vi "GetFilePathAndDate.vi"(8 "error in (no error)":errorcluster, 9 "String":string, 10 "Index":i32, 11 "Path":path) -> (0 "error out":errorcluster, 2 "creation date":u32, 3 "file out":path)   [LabVIEW 2015]
uses:
  <userlib>/_OpenG.lib/file/file.llb/File Info Record__ogtk.ctl
panel:
  out "file info":T1={"type"="????", "creator"="????", "permissions"=438, "data size"=5687, "res size"=0, "creation date"=3188231670, "modification date"=3188232972, "bFolder"=FALSE, "bInvisible"=FALSE, "location"={"vertical"=0, "horizontal"=0}, "owner"="", "group"=""} {"modification date" format="%<%H:%M:%S\n%m/%d/%Y>T"; "creation date" format="%<%H:%M:%S\n%m/%d/%Y>T"; "permissions" format="%.0x"}
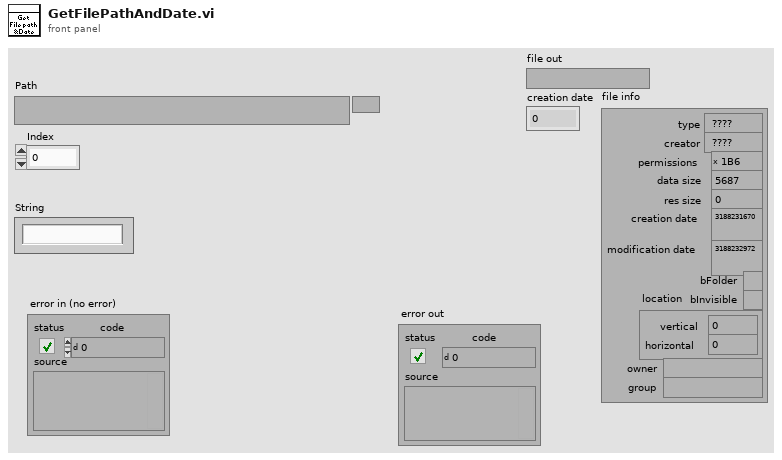
[diagram p1: front panel]
types:
  T1 = typedef "File Info Record__ogtk.ctl" = cluster{"type":string, "creator":string, "permissions":i32, "data size":i32, "res size":i32, "creation date":u32, "modification date":u32, "bFolder":bool, "bInvisible":bool, "location":cluster{"vertical":i16, "horizontal":i16}, "owner":string, "group":string}
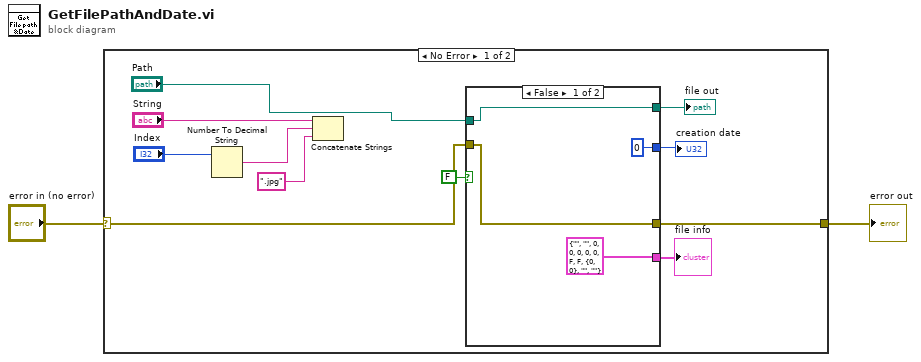
[diagram p0: block diagram]
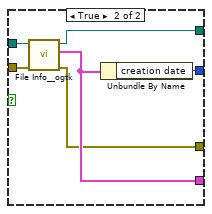
[diagram p2: hidden frame]
diagram:
  n1 = case shown="No Error" "error in (no error)" {
    selector: "error in (no error)" -> [w7 w24]
    tunnel: [w6 w24] -> w1
    frame No Error {
      n2 = Number To Decimal String(number="Index") -> (decimal integer string=w12:string)  [unwired: 1 in]
      n3 = Concatenate Strings("String", w12, ".jpg" ("string")) -> ()  [unwired: 1 out]
      n4 = case shown="False" FALSE {
        tunnel: [T1 {"type"="", "creator"="", "permissions"=0, "data size"=0, "res size"=0, "creation date"=0, "modification date"=0, "bFolder"=FALSE, "bInvisible"=FALSE, "location"={"vertical"=0, "horizontal"=0}, "owner"="", "group"=""} ("file info") w23] -> w10
        tunnel: [u32 0 ("creation date") w22] -> w8
        tunnel: w7 -> [w16 w21]
        tunnel: [w16 w20] -> w6
        tunnel: "Path" -> [w17 w19]
        tunnel: [w17 w18] -> w5
        frame False {
        }
        frame True {
          n5 = call <userlib>:"File Info__ogtk.vi"("error in (no error)"=w21, "file"=w19) -> ("error out"=w20:errorcluster, "file info"=w23:T1, "file out"=w18:path)  [unwired: 4 in]
          n6 = Unbundle By Name(w23) -> ("creation date"=w22:u32)
        }
      }
      "file out" <- w5
      "creation date" <- w8
      "file info" <- w10
    }
    frame Error {
    }
  }
  "error out" <- w1
